vi "5 - Write to File (Solution).vi"() -> ()   [LabVIEW 2012]
panel:
  out "Alarm Output":bool
  in  "Alarm Level":dbl=26.0
  out "Temperature Data":dynamicdata(graph)
  in  "stop":bool
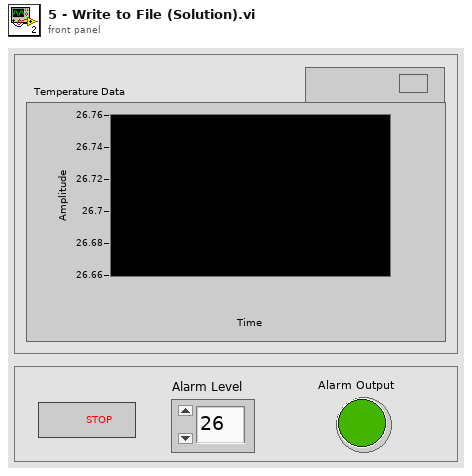
[diagram p1: front panel]
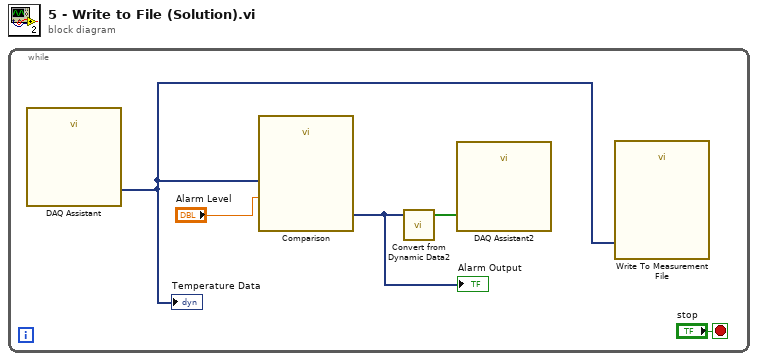
[diagram p0: block diagram]
diagram:
  n1 = while {
    stop <- "stop" stop-if-true
    n2 = call "DAQ Assistant"() -> ("data"=w3:dynamicdata)  [unwired: 16 in, 3 out]
    "Temperature Data" <- w3
    n3 = call "Comparison"("Operand 2"="Alarm Level", "Operand 1"=w3) -> ("Result"=w4:dynamicdata)  [unwired: 1 in, 8 out]
    "Alarm Output" <- w4
    n4 = call "Convert from Dynamic Data2"("Dynamic Data Type"=w4) -> ("Array"=w5:bool[])  [unwired: 3 out]
    n5 = call "DAQ Assistant2"("data"=w5) -> ()  [unwired: 4 in, 15 out]
    n6 = call "Write To Measurement File"("Signals"=w3) -> ()  [unwired: 16 in, 3 out]
  }
